vi "atMonochromator_logEvent_MonochromatorConnected.vi"(8 "error in (no error)":errorcluster, 11 "logevent_MonochromatorConnected_Ctl":T1) -> (0 "error out":errorcluster, 2 "function return":i32, 3 "logevent_MonochromatorConnected_Ctl out":T1)   [LabVIEW 2016, in "SALLV_atMonochromator.lvlib"]
doc: "int atMonochromator_shm_logEvent_MonochromatorConnectedLV(atMonochromator_logevent_MonochromatorConnectedLV *logevent_MonochromatorConnected_Ctl );"
uses:
  SALLV_atMonochromator.lvlib
  DataTypes/logevent_MonochromatorConnected.ctl
  SALLV_atMonochromator.so
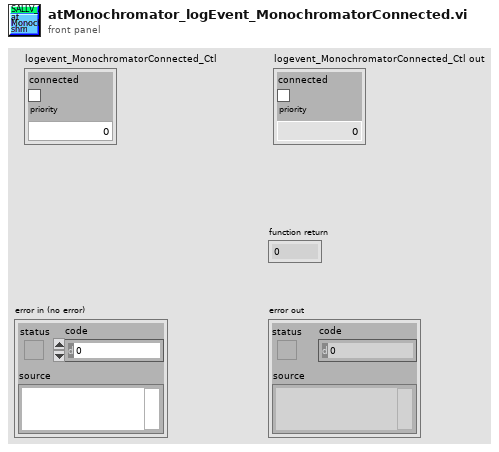
[diagram p1: front panel]
types:
  T1 = typedef "SALLV_atMonochromator.lvlib/logevent_MonochromatorConnected.ctl" = cluster{"connected":bool, "priority":i32}
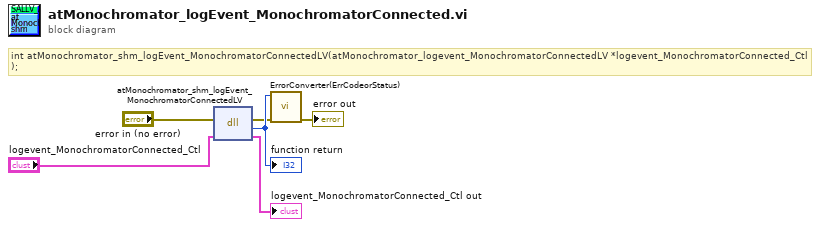
[diagram p0: block diagram]
diagram:
  # "int atMonochromator_shm_logEvent_MonochromatorConnectedLV(atMonochromator_logevent_MonochromatorConnectedLV *logevent_MonochromatorConnected_Ctl );"
  n1 = dll-call lib="home/andres/Desktop/SAL_atMonochromator/SALLV_atMonochromator.*" fn="atMonochromator_shm_logEvent_MonochromatorConnectedLV"(error in="error in (no error)", "logevent_MonochromatorConnected_Ctl"="logevent_MonochromatorConnected_Ctl") -> (error out=w2:errorcluster, w6:i32, "logevent_MonochromatorConnected_Ctl"=→"logevent_MonochromatorConnected_Ctl out":T1)  [unwired: 2 in, 1 out]
  "function return" <- w6
  n2 = call "ErrorConverter(ErrCodeorStatus).vi"("error in (no error)"=w2, "error code"=w6) -> ("error out"=→"error out":errorcluster)  [unwired: 9 in]
